vi "Joystick disconnect detect.vi"() -> ()   [LabVIEW 2015]
uses:
  <vilib>/Utility/inputDevices.llb/joystickAcquire.vi
  <vilib>/Utility/inputDevices.llb/closeJoystick.vi
panel:
  out "Boolean":bool
  in  "stop":bool
  out "button 1":bool
  out "Numeric":i32
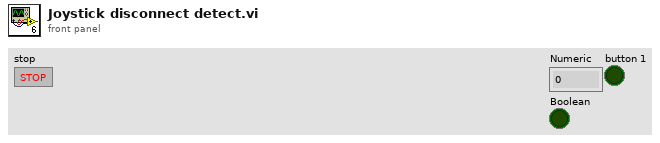
[diagram p1: front panel]
types:
  T1 = cluster{"axes total":u32, "buttons total":u32, "pov total":u32, "device name":string}[]
  T2 = cluster{"button 1":bool, "button 2":bool, "button 3":bool, "button 4":bool, "button 5":bool, "button 6":bool, "button 7":bool, "button 8":bool, "button 9":bool, "button 10":bool, "button 11":bool, "button 12":bool, "button 13":bool, "button 14":bool, "button 15":bool, "button 16":bool, "button 17":bool, "button 18":bool, "button 19":bool, "button 20":bool, "button 21":bool, "button 22":bool, "button 23":bool, "button 24":bool, "button 25":bool, "button 26":bool, "button 27":bool, "button 28":bool, "button 29":bool, "button 30":bool, "button 31":bool, "button 32":bool}
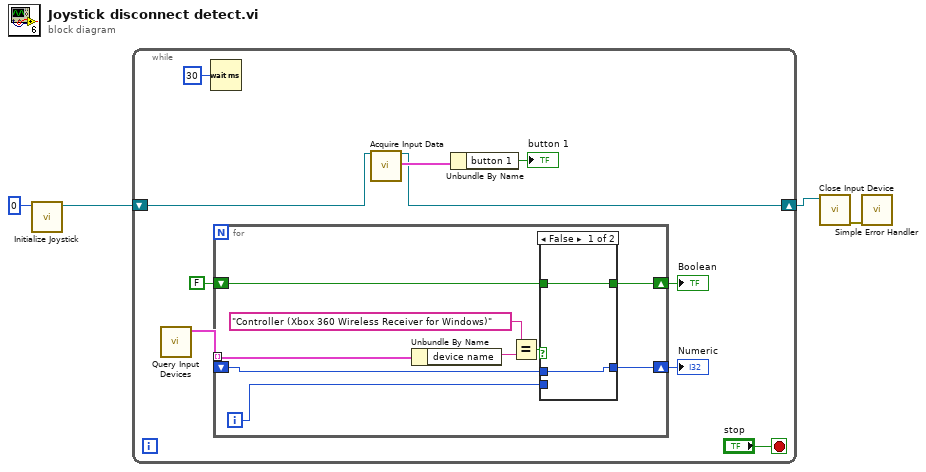
[diagram p0: block diagram]
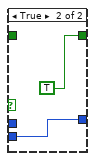
[diagram p2: hidden frame]
diagram:
  n1 = call <vilib>:"Initialize Joystick.vi"("device index"=0) -> ("device ID"=w2:refnum<k1>)  [unwired: 1 in, 9 out]
  n2 = while {
    shift-right: [w7] -> w1
    shift-left: w2 -> [w8]
    stop <- "stop" stop-if-true
    n3 = call <vilib>:"Query Input Devices.vi"() -> ("joystick info"=w14:T1)  [unwired: 1 in, 10 out]
    n4 = Wait (ms)(milliseconds to wait=u32 30) -> ()  [unwired: 1 out]
    n5 = for {
      tunnel: w14 -> [w23] mode=indexing
      shift-right: [w19] -> w13
      shift-left: _ -> [w17]
      shift-right: [w16] -> w5
      shift-left: FALSE -> [w15]
      i -> [w18]
      n6 = Unbundle By Name(w23) -> ("device name"=w22:string)
      n7 = Equal?(x="Controller (Xbox 360 Wireless Receiver for Windows)", y=w22) -> (x = y?=w20:bool)
      n8 = case shown="False" w20 {
        tunnel: [w25 w27] -> w19
        tunnel: w18 -> [_ w27]
        tunnel: w17 -> [w25 _]
        tunnel: [w24 TRUE] -> w16
        tunnel: w15 -> [w24 _]
        frame False {
        }
        frame True {
        }
      }
    }
    "Numeric" <- w13
    "Boolean" <- w5
    n9 = call-poly <vilib>:"Acquire Input Data.vi"("device ID"=w8) -> ("device ID"=w7:refnum<k1>, "button info"=w10:T2)  [unwired: 14 in, 3 out]
    n10 = Unbundle By Name(w10) -> ("button 1"=→"button 1":bool)
  }
  n11 = call-poly <vilib>:"Close Input Device.vi"("device ID"=w1) -> ("error out"=w4:errorcluster)  [unwired: 1 in, 8 out]
  n12 = call <vilib>:"Simple Error Handler.vi"("error in (no error)"=w4) -> ()  [unwired: 1 in, 8 out]
